vi "temperature_from_string.vi"(1 "data in":string) -> (0 "temperatura":dbl)   [LabVIEW 2021]
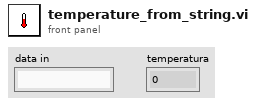
[diagram p1: front panel]
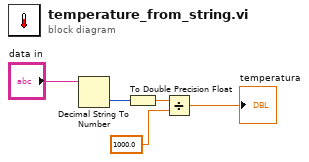
[diagram p0: block diagram]
diagram:
  n1 = Decimal String To Number(string="data in") -> (number=w4:i32)  [unwired: 2 in, 1 out]
  n2 = To Double Precision Float(number=w4) -> (double precision float=w3:dbl)
  n3 = Divide(x=w3, y=1000.0) -> (x/y=→"temperatura":dbl)
